vi "Process CSV.vi"() -> ()   [LabVIEW 2018, in "Stage Actor.lvlib" / "Stage.lvclass"]
uses:
  Stage.lvclass
  <vilib>/Utility/file.llb/Read Delimited Spreadsheet (string).vi
  Stage Actor.lvlib
panel:
  in  "Stage Actor":refnum<class "Stage.lvclass">
  in  "Read Coordinates from CSV":path
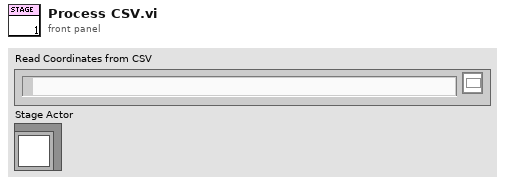
[diagram p1: front panel]
types:
  T1 = cluster{"XYZ":dbl[][], "Theta Phi":dbl[][], "Current Tool":i16[], "Speed":dbl[], "Feeder State":bool[]}
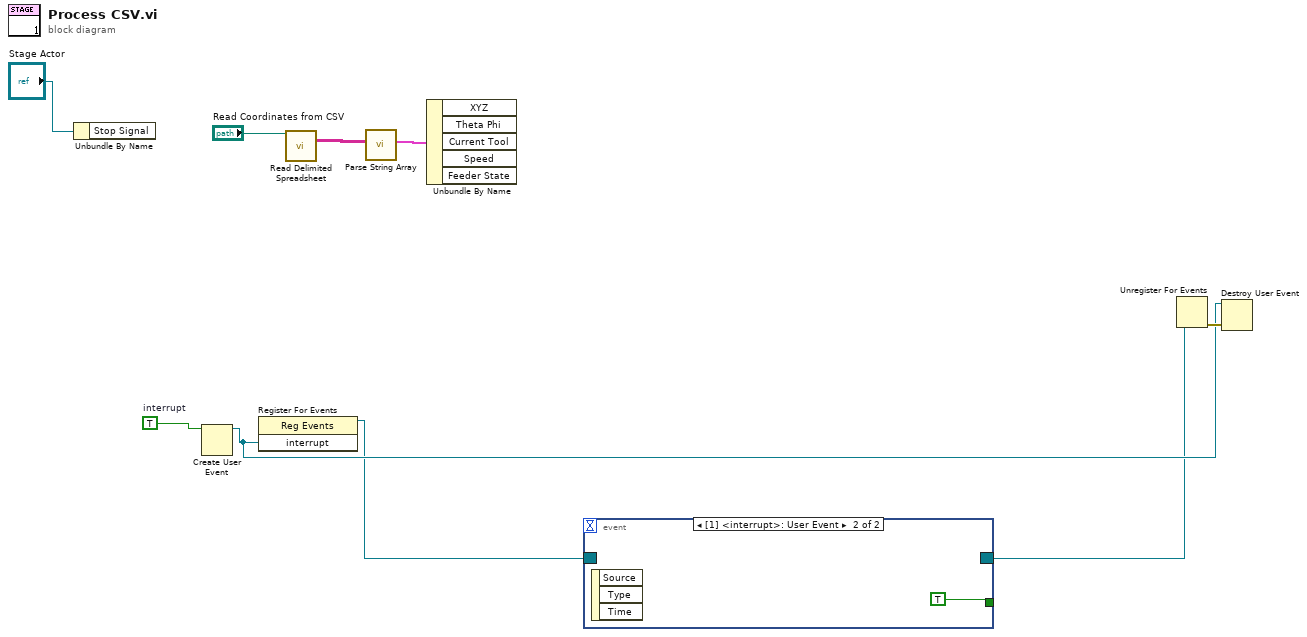
[diagram p0: block diagram]
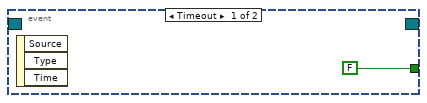
[diagram p2: hidden frame]
diagram:
  w9 = TRUE  # interrupt
  n1 = Unbundle By Name("Stage Actor") -> ()  [unwired: 1 out]
  n2 = Create User Event(user event datatype=w9) -> (user event=w7:refnum<user-event>)  [unwired: 1 in, 1 out]
  n3 = register-events(w7) -> (reference out=w3:refnum<event-registration>)  [unwired: 2 in, 1 out]
  n4 = call-poly <vilib>:"Read Delimited Spreadsheet.vi"("file path (dialog if empty)"="Read Coordinates from CSV") -> ("all rows"=w5:string[][])  [unwired: 9 in, 5 out]
  n5 = call "Parse String Array.vi"("String XYZ"=w5) -> ("Line Data"=w1:T1)  [unwired: 9 in, 1 out]
  n6 = Unbundle By Name(w1) -> ()  [unwired: 5 out]
  n7 = event shown="[1] <interrupt>: User Event" {
    selector: w3 -> [_ _]
    dyn-events: [_ _] -> w2
    timeout: _ -> [_ _]
    tunnel: [FALSE TRUE] -> _
    event Timeout {
      n8 = event-data() -> ()  [unwired: 1 in, 3 out]
    }
    event User Event {
      n9 = event-data() -> ()  [unwired: 1 in, 3 out]
    }
  }
  n10 = Unregister For Events(event registration refnum=w2) -> (error out=w8:errorcluster)  [unwired: 1 in]
  n11 = Destroy User Event(user event=w7, error in=w8) -> ()  [unwired: 1 out]
